vi "Tool RS232 testS3.vi"(8 "error in (no error)":errorcluster, 10 "VISA resource name":refnum<visa-resource-name>="COM3", 11 "action":u16(ring) items=["INITIAL", "RESET", "FORMAT", "PROGRAM1", "PROGRAM2", "FSKSCAN", "ASKSCAN"]) -> (0 "error out":errorcluster, 3 "receive string":string)   [LabVIEW 2019]
panel:
  out "read string":string
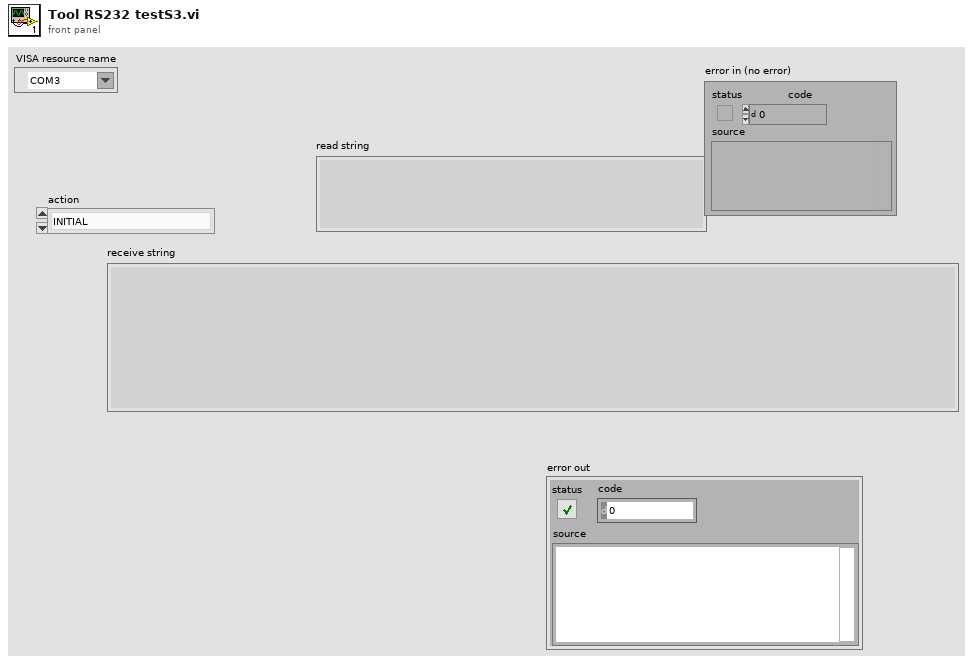
[diagram p1: front panel]
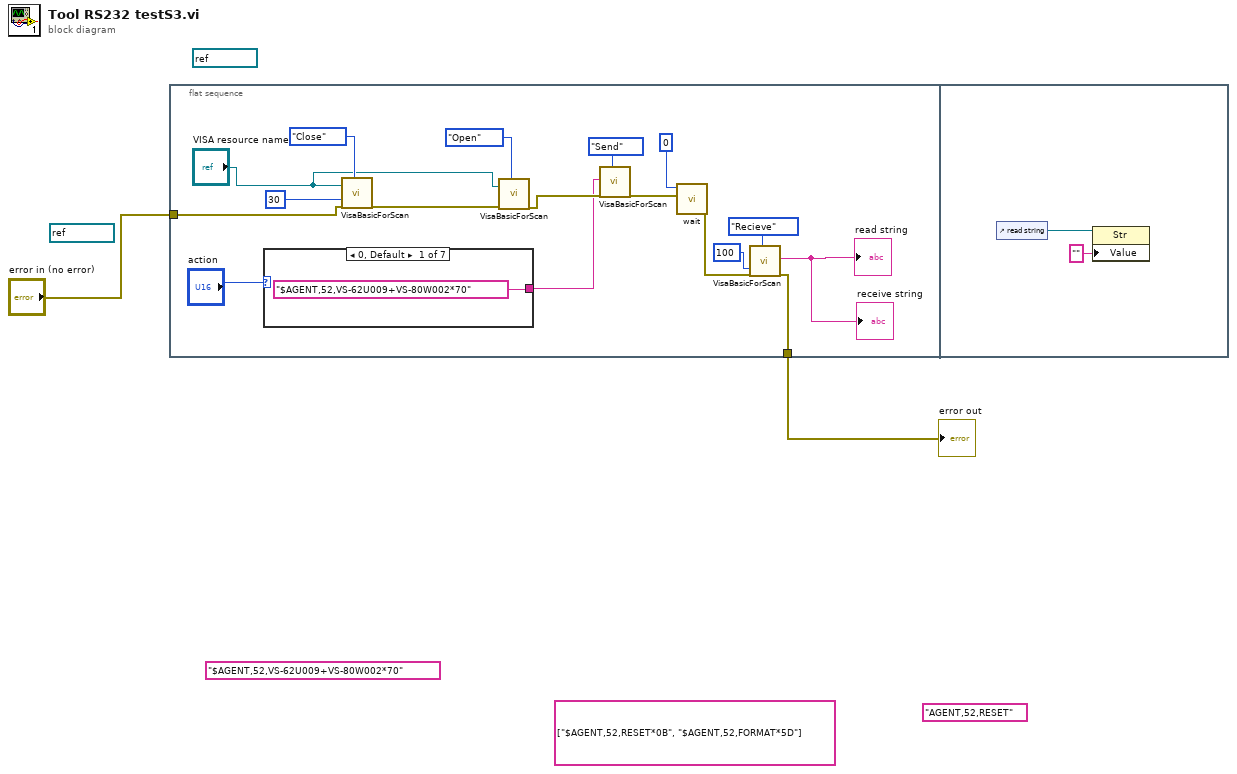
[diagram p0: block diagram]
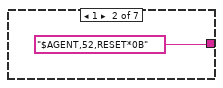
[diagram p2: hidden frame]
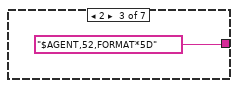
[diagram p3: hidden frame]
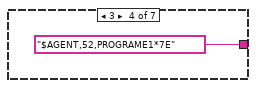
[diagram p4: hidden frame]
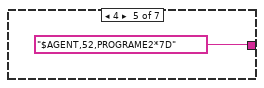
[diagram p5: hidden frame]
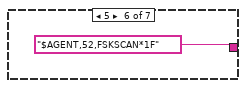
[diagram p6: hidden frame]
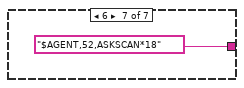
[diagram p7: hidden frame]
diagram:
  (unwired) refnum<visa-resource-name> "COM3" ("VISA resource name")
  (unwired) refnum<visa-resource-name> "COM3" ("VISA resource name")
  (unwired) "AGENT,52,RESET"
  (unwired) "$AGENT,52,VS-62U009+VS-80W002*70" ("Cmd 2")
  (unwired) string[] ["$AGENT,52,RESET*0B", "$AGENT,52,FORMAT*5D"]
  n1 = flat-sequence {
    tunnel: [w5] -> w2
    tunnel: "error in (no error)" -> [w3]
    frame #0 {
      n2 = case shown="0, Default" "action" {
        tunnel: ["$AGENT,52,VS-62U009+VS-80W002*70" ("Cmd 2") "$AGENT,52,RESET*0B" ("Cmd 2") "$AGENT,52,FORMAT*5D" ("Cmd 2") "$AGENT,52,PROGRAME1*7E" ("Cmd 2") "$AGENT,52,PROGRAME2*7D" ("Cmd 2") "$AGENT,52,FSKSCAN*1F" ("Cmd 2") "$AGENT,52,ASKSCAN*18" ("Cmd 2")] -> w9
        frame 0, Default {
        }
        frame 1 {
        }
        frame 2 {
        }
        frame 3 {
        }
        frame 4 {
        }
        frame 5 {
        }
        frame 6 {
        }
      }
      n3 = call "VisaBasicForScan.vi"("VISA resource name"="VISA resource name", "Time(0.1)"=30, "error in (no error)"=w3, "VisaAction"=enum16{"Open", "Send", "Recieve", "Close"}."Close") -> ("error out"=w16:errorcluster)  [unwired: 14 in, 1 out]
      n4 = call "VisaBasicForScan.vi"("VISA resource name"="VISA resource name", "error in (no error)"=w16, "VisaAction"=enum16{"Open", "Send", "Recieve", "Close"}."Open") -> ("error out"=w14:errorcluster)  [unwired: 15 in, 1 out]
      n5 = call "VisaBasicForScan.vi"("Cmd"=w9, "error in (no error)"=w14, "VisaAction"=enum16{"Open", "Send", "Recieve", "Close"}."Send") -> ("error out"=w7:errorcluster)  [unwired: 15 in, 1 out]
      n6 = call "wait.vi"("error in"=w7, "wait(ms)"=u32 0) -> ("error out"=w6:errorcluster)  [unwired: 9 in]
      n7 = call "VisaBasicForScan.vi"("Time(0.1)"=u32 100, "error in (no error)"=w6, "VisaAction"=enum16{"Open", "Send", "Recieve", "Close"}."Recieve") -> ("read string"=→"read string" →"receive string":string, "error out"=w5:errorcluster)  [unwired: 15 in]
    }
    frame #1 {
      n8 = control-ref of="read string"() -> (w28:refnum<vi>)
      n9 = property class="Str"(reference=w28, "Value"="") -> ()  [unwired: 1 in, 2 out]
    }
  }
  "error out" <- w2
